vi "Obtain Request Events.vi"(8 "error in (no error)":errorcluster, 10 "Create New?":bool) -> (0 "error out":errorcluster, 2 "Power Supply Request Events":T1)   [LabVIEW 2025, in "Power Supply.lvlib"]
doc: "This VI Obtains/Creates the Requests events that will be used for other modules to communicate with the module that owns this VI. These Requests events will be accessed only via Public API methods for this module.\n\n<b>NOTE</b>: The contents of this VI are automatically generated and modified by the <b>Tools > Delacor > DQMH</b> utilities. Consider using those utilities instead of making your own modifications to this VI.\n_____\nBased on Delacor QMH Project Template 3.1.0.34."
uses:
  Power Supply.lvlib
  Request Events--cluster.ctl
  Stop Argument--cluster.ctl
  Get Module Execution Status Argument--cluster.ctl
  Show Diagram Argument--cluster.ctl
  Hide Panel Argument--cluster.ctl
  Show Panel Argument--cluster.ctl
  <vilib>/MGI/Panel Manager/Panel/Panel/Panel.lvclass
  Change Panel Argument--cluster.ctl
  Set Current SP Argument--cluster.ctl
  Set Voltage SP Argument--cluster.ctl
  Set Power SP Argument--cluster.ctl
  Set Power Supply Plugin Argument--cluster.ctl
  DC Output--enum.ctl
  Set DC Output Argument--cluster.ctl
  Sleep Connection Helper Loop Argument--cluster.ctl
  Connect Argument--cluster.ctl
  Disconnect Argument--cluster.ctl
  Function Generator State--cluster.ctl
  Set Function Generator State Argument--cluster.ctl
  Wake Connection Helper Loop Argument--cluster.ctl
  Set DC Current SP Argument--cluster.ctl
  Set DC Voltage SP Argument--cluster.ctl
  Set DC Power SP Argument--cluster.ctl
  Set DC Output SP Argument--cluster.ctl
  Function Generator Parameters--cluster.ctl
  Set Function Generator Parameters Argument--cluster.ctl
  Set Function Generator Parameters SP Argument--cluster.ctl
  Set Function Generator State SP Argument--cluster.ctl
panel:
  # "NOTE: The contents of this VI are automatically generated and modified by the Tools > Delacor > DQMH utilities. Consider using those utilities instead of making your own modifications to this VI."
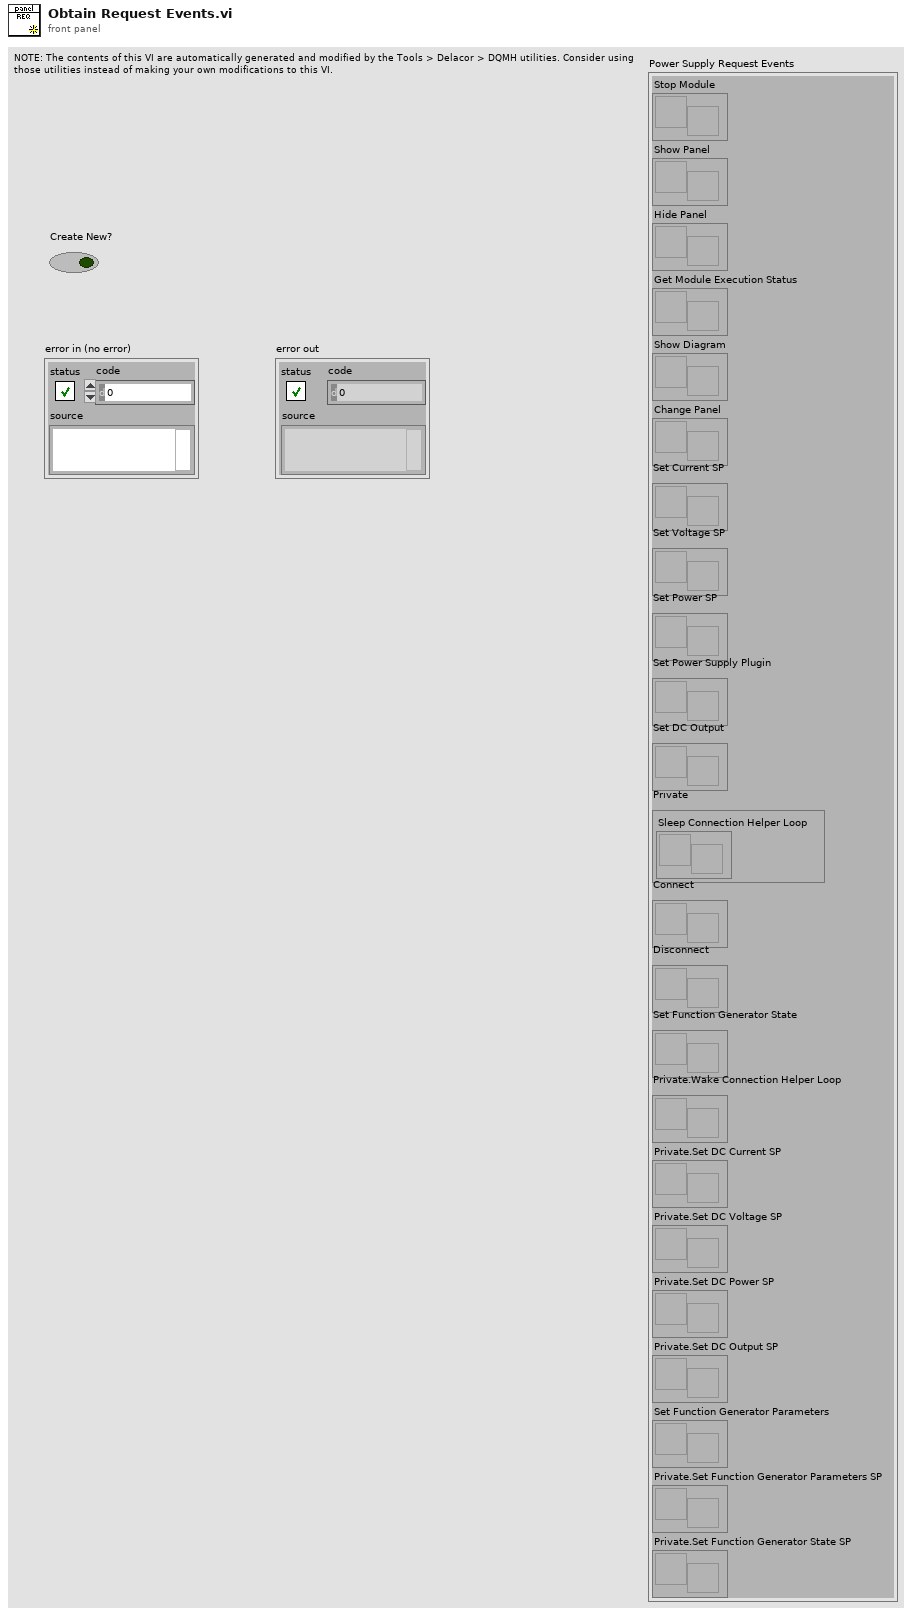
[diagram p1: front panel]
types:
  T1 = typedef "Power Supply.lvlib/Request Events--cluster.ctl" = cluster{"Stop Module":refnum<user-event>, "Show Panel":refnum<user-event>, "Hide Panel":refnum<user-event>, "Get Module Execution Status":refnum<user-event>, "Show Diagram":refnum<user-event>, "Change Panel":refnum<user-event>, "Set Current SP":refnum<user-event>, "Set Voltage SP":refnum<user-event>, "Set Power SP":refnum<user-event>, "Set Power Supply Plugin":refnum<user-event>, "Set DC Output":refnum<user-event>, "Private":cluster{"Sleep Connection Helper Loop":refnum<user-event>}, "Connect":refnum<user-event>, "Disconnect":refnum<user-event>, "Set Function Generator State":refnum<user-event>, "Private.Wake Connection Helper Loop":refnum<user-event>, "Private.Set DC Current SP":refnum<user-event>, "Private.Set DC Voltage SP":refnum<user-event>, "Private.Set DC Power SP":refnum<user-event>, "Private.Set DC Output SP":refnum<user-event>, "Set Function Generator Parameters":refnum<user-event>, "Private.Set Function Generator Parameters SP":refnum<user-event>, "Private.Set Function Generator State SP":refnum<user-event>}
  T2 = typedef "Power Supply.lvlib/Set Function Generator State SP Argument--cluster.ctl" = cluster{"Function Generator State":T3}
  T3 = typedef "Power Supply.lvlib/Function Generator State--cluster.ctl" = enum16{"DISABLE", "ENABLE"}
  T4 = typedef "Power Supply.lvlib/Set Function Generator Parameters SP Argument--cluster.ctl" = cluster{"Function Generator":T5}
  T5 = typedef "Power Supply.lvlib/Function Generator Parameters--cluster.ctl" = cluster{"Us_AC":sgl, "Ue_AC":sgl, "fs_Hz":sgl, "fe_Hz ":sgl, "angle_deg ":sgl, "Us_DC ":sgl, "Ue_DC":sgl, "seq_time_us":sgl}
  T6 = typedef "Power Supply.lvlib/Set Function Generator Parameters Argument--cluster.ctl" = cluster{"Function Generator":T5}
  T7 = typedef "Power Supply.lvlib/Set DC Output SP Argument--cluster.ctl" = cluster{"DC Ouput":T8}
  T8 = typedef "Power Supply.lvlib/DC Output--enum.ctl" = enum16{"OFF", "ON"}
  T9 = typedef "Power Supply.lvlib/Set DC Power SP Argument--cluster.ctl" = cluster{"DC Power SP [W]":dbl}
  T10 = typedef "Power Supply.lvlib/Set DC Voltage SP Argument--cluster.ctl" = cluster{"DC Voltage SP [V]":dbl}
  T11 = typedef "Power Supply.lvlib/Set DC Current SP Argument--cluster.ctl" = cluster{"DC Current [A]":dbl}
  T12 = typedef "Power Supply.lvlib/Wake Connection Helper Loop Argument--cluster.ctl" = cluster{"Boolean":bool}
  T13 = typedef "Power Supply.lvlib/Set Function Generator State Argument--cluster.ctl" = cluster{"Function Generator State":T3}
  T14 = typedef "Power Supply.lvlib/Disconnect Argument--cluster.ctl" = cluster{"Boolean":bool}
  T15 = typedef "Power Supply.lvlib/Connect Argument--cluster.ctl" = cluster{"Boolean":bool}
  T16 = typedef "Power Supply.lvlib/Sleep Connection Helper Loop Argument--cluster.ctl" = cluster{"Boolean":bool}
  T17 = typedef "Power Supply.lvlib/Set DC Output Argument--cluster.ctl" = cluster{"DC Ouput":T8}
  T18 = typedef "Power Supply.lvlib/Set Power Supply Plugin Argument--cluster.ctl" = cluster{"Plugin File Path":path}
  T19 = typedef "Power Supply.lvlib/Set Power SP Argument--cluster.ctl" = cluster{"Power [W]":dbl}
  T20 = typedef "Power Supply.lvlib/Set Voltage SP Argument--cluster.ctl" = cluster{"Voltage SP [V]":dbl}
  T21 = typedef "Power Supply.lvlib/Set Current SP Argument--cluster.ctl" = cluster{"Current SP [A]":dbl}
  T22 = typedef "Power Supply.lvlib/Change Panel Argument--cluster.ctl" = cluster{"New Panel":refnum<class "Panel.lvclass">}
  T23 = typedef "Power Supply.lvlib/Hide Panel Argument--cluster.ctl" = cluster{"Hide Panel?":bool}
  T24 = typedef "Power Supply.lvlib/Show Panel Argument--cluster.ctl" = cluster{"Show Panel?":bool}
  T25 = typedef "Power Supply.lvlib/Show Diagram Argument--cluster.ctl" = cluster{"Debug?":bool}
  T26 = typedef "Power Supply.lvlib/Get Module Execution Status Argument--cluster.ctl" = cluster{"Running?":bool}
  T27 = typedef "Power Supply.lvlib/Stop Argument--cluster.ctl" = cluster{"Origin":string, "Exit via Stop Module Req?":bool, "Wait for Module to stop?":bool}
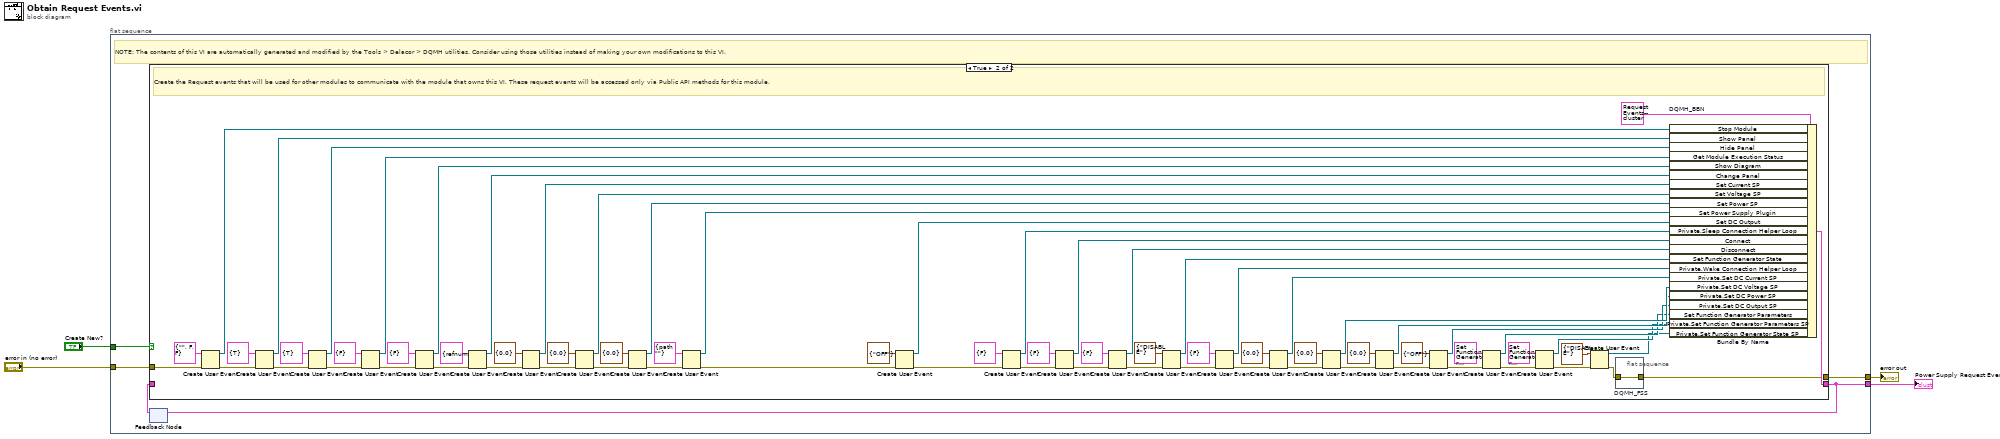
[diagram p0: block diagram]
diagram:
  n1 = flat-sequence {
    tunnel: [w9] -> w4
    tunnel: "error in (no error)" -> [w8]
    tunnel: [w6] -> w2
    tunnel: "Create New?" -> [w5]
    frame #0 {
      # "NOTE: The contents of this VI are automatically generated and modified by the Tools > Delacor > DQMH utilities. Consider using those utilities instead of making your own modifications to this VI."
      n2 = feedback #1() -> (w7:T1)  [unwired: 1 in]
      n3 = case shown="True" w5 {
        tunnel: [w10 w74] -> w9
        tunnel: w8 -> [w10 w84]
        tunnel: [w11 w81] -> w6
        tunnel: w7 -> [w11 _]
        frame False {
          # "Obtain the Request events that were created in a previous call to this VI."
        }
        frame True {
          # "Create the Request events that will be used for other modules to communicate with the module that owns this VI. These request events will be accessed only via Public API methods for this module."
          n4 = Create User Event(user event datatype=T27 {"Origin"="", "Exit via Stop Module Req?"=FALSE, "Wait for Module to stop?"=FALSE} ("Stop Argument"), error in=w84) -> (user event=w82:refnum<user-event>, error out=w79:errorcluster)
          n5 = Create User Event(user event datatype=T24 {"Show Panel?"=TRUE} ("Show Panel Argument"), error in=w79) -> (user event=w78:refnum<user-event>, error out=w77:errorcluster)
          n6 = Create User Event(user event datatype=T23 {"Hide Panel?"=TRUE} ("Hide Panel Argument"), error in=w77) -> (user event=w76:refnum<user-event>, error out=w75:errorcluster)
          n7 = Create User Event(user event datatype=T26 {"Running?"=FALSE} ("Get Module Execution Status Argument"), error in=w75) -> (user event=w72:refnum<user-event>, error out=w73:errorcluster)
          n8 = Create User Event(user event datatype=T25 {"Debug?"=FALSE} ("Show Diagram Argument"), error in=w73) -> (user event=w69:refnum<user-event>, error out=w70:errorcluster)
          n9 = Create User Event(user event datatype=T22 {"New Panel"=refnum} ("Change Panel Argument"), error in=w70) -> (user event=w64:refnum<user-event>, error out=w65:errorcluster)
          n10 = Create User Event(user event datatype=T21 {"Current SP [A]"=0.0} ("Set Current SP Argument"), error in=w65) -> (user event=w61:refnum<user-event>, error out=w62:errorcluster)
          n11 = Create User Event(user event datatype=T20 {"Voltage SP [V]"=0.0} ("Set Voltage SP Argument"), error in=w62) -> (user event=w58:refnum<user-event>, error out=w59:errorcluster)
          n12 = Create User Event(user event datatype=T19 {"Power [W]"=0.0} ("Set Power SP Argument"), error in=w59) -> (user event=w55:refnum<user-event>, error out=w56:errorcluster)
          n13 = Create User Event(user event datatype=T18 {"Plugin File Path"=path ""} ("Set Power Supply Plugin Argument"), error in=w56) -> (user event=w52:refnum<user-event>, error out=w53:errorcluster)
          n14 = Create User Event(user event datatype=T17 {"DC Ouput"=enum."OFF"} ("Set DC Output Argument"), error in=w53) -> (user event=w49:refnum<user-event>, error out=w50:errorcluster)
          n15 = Create User Event(user event datatype=T16 {"Boolean"=FALSE} ("Sleep Connection Helper Loop Argument"), error in=w50) -> (user event=w46:refnum<user-event>, error out=w47:errorcluster)
          n16 = Create User Event(user event datatype=T15 {"Boolean"=FALSE} ("Connect Argument"), error in=w47) -> (user event=w43:refnum<user-event>, error out=w44:errorcluster)
          n17 = Create User Event(user event datatype=T14 {"Boolean"=FALSE} ("Disconnect Argument"), error in=w44) -> (user event=w40:refnum<user-event>, error out=w41:errorcluster)
          n18 = Create User Event(user event datatype=T13 {"Function Generator State"=enum."DISABLE"} ("Set Function Generator State Argument"), error in=w41) -> (user event=w37:refnum<user-event>, error out=w38:errorcluster)
          n19 = Create User Event(user event datatype=T12 {"Boolean"=FALSE} ("Wake Connection Helper Loop Argument"), error in=w38) -> (user event=w34:refnum<user-event>, error out=w35:errorcluster)
          n20 = Create User Event(user event datatype=T11 {"DC Current [A]"=0.0} ("Set DC Current SP Argument"), error in=w35) -> (user event=w31:refnum<user-event>, error out=w32:errorcluster)
          n21 = Create User Event(user event datatype=T10 {"DC Voltage SP [V]"=0.0} ("Set DC Voltage SP Argument"), error in=w32) -> (user event=w28:refnum<user-event>, error out=w29:errorcluster)
          n22 = Create User Event(user event datatype=T9 {"DC Power SP [W]"=0.0} ("Set DC Power SP Argument"), error in=w29) -> (user event=w25:refnum<user-event>, error out=w26:errorcluster)
          n23 = Create User Event(user event datatype=T7 {"DC Ouput"=enum."OFF"} ("Set DC Output SP Argument"), error in=w26) -> (user event=w22:refnum<user-event>, error out=w23:errorcluster)
          n24 = Create User Event(user event datatype=T6 {"Function Generator"={"Us_AC"=0.0, "Ue_AC"=0.0, "fs_Hz"=0.0, "fe_Hz "=0.0, "angle_deg "=0.0, "Us_DC "=0.0, "Ue_DC"=0.0, "seq_time_us"=0.0}} ("Set Function Generator Parameters Argument"), error in=w23) -> (user event=w19:refnum<user-event>, error out=w20:errorcluster)
          n25 = Create User Event(user event datatype=T4 {"Function Generator"={"Us_AC"=0.0, "Ue_AC"=0.0, "fs_Hz"=0.0, "fe_Hz "=0.0, "angle_deg "=0.0, "Us_DC "=0.0, "Ue_DC"=0.0, "seq_time_us"=0.0}} ("Set Function Generator Parameters SP Argument"), error in=w20) -> (user event=w16:refnum<user-event>, error out=w17:errorcluster)
          n26 = Create User Event(user event datatype=T2 {"Function Generator State"=enum."DISABLE"} ("Set Function Generator State SP Argument"), error in=w17) -> (user event=w13:refnum<user-event>, error out=w14:errorcluster)
          n27 = flat-sequence "DQMH_FSS" {
            tunnel: w14 -> [w85]
            tunnel: [w85] -> w74
            frame #0 {
            }
          }
          n28 = Bundle By Name "DQMH_BBN"(cluster=T1 {"Stop Module"=refnum, "Show Panel"=refnum, "Hide Panel"=refnum, "Get Module Execution Status"=refnum, "Show Diagram"=refnum, "Change Panel"=refnum, "Set Current SP"=refnum, "Set Voltage SP"=refnum, "Set Power SP"=refnum, "Set Power Supply Plugin"=refnum, "Set DC Output"=refnum, "Private"={"Sleep Connection Helper Loop"=refnum}, "Connect"=refnum, "Disconnect"=refnum, "Set Function Generator State"=refnum, "Private.Wake Connection Helper Loop"=refnum, "Private.Set DC Current SP"=refnum, "Private.Set DC Voltage SP"=refnum, "Private.Set DC Power SP"=refnum, "Private.Set DC Output SP"=refnum, "Set Function Generator Parameters"=refnum, "Private.Set Function Generator Parameters SP"=refnum, "Private.Set Function Generator State SP"=refnum} ("output cluster"), "Stop Module"=w82, "Show Panel"=w78, "Hide Panel"=w76, "Get Module Execution Status"=w72, "Show Diagram"=w69, "Change Panel"=w64, "Set Current SP"=w61, "Set Voltage SP"=w58, "Set Power SP"=w55, "Set Power Supply Plugin"=w52, "Set DC Output"=w49, "Private.Sleep Connection Helper Loop"=w46, "Connect"=w43, "Disconnect"=w40, "Set Function Generator State"=w37, "Private.Wake Connection Helper Loop"=w34, "Private.Set DC Current SP"=w31, "Private.Set DC Voltage SP"=w28, "Private.Set DC Power SP"=w25, "Private.Set DC Output SP"=w22, "Set Function Generator Parameters"=w19, "Private.Set Function Generator Parameters SP"=w16, "Private.Set Function Generator State SP"=w13) -> (w81:T1)
        }
      }
      n29 = feedback-in #1(w6) -> ()
    }
  }
  "Power Supply Request Events" <- w2
  "error out" <- w4
